vi "check interlock status.vi"(11 "Interlocks":T1) -> (3 "interlocksOK":bool)   [LabVIEW 2018]
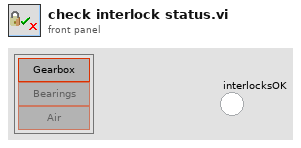
[diagram p1: front panel]
types:
  T1 = cluster{"gearboxOil":bool, "bearingOil":bool, "gearboxAir":bool}
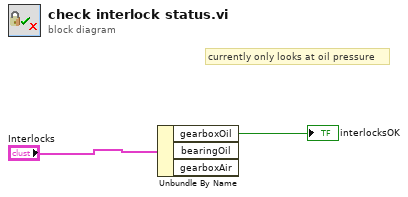
[diagram p0: block diagram]
diagram:
  # "currently only looks at oil pressure"
  n1 = Unbundle By Name("Interlocks") -> ("gearboxOil"=→"interlocksOK":bool)  [unwired: 2 out]
